vi "Read Single.vi"(0 "RS232 Port In":refnum<visa-resource-name>="COM12", 1 "Sensor Address In":string="0", 4 "Measurement Type In (Normal)":i32(ring) items=["Normal", "Concurrent", "Continuous"], 5 "CRC (False)":bool, 6 "Parameter In (0)":i32(ring) items=["0", "1", "2", "3", "4", "5", "6", "7", "8", "9"], 7 "Error In (No Error)":errorcluster, 10 "Initialize/close":bool) -> (20 "RS232 Port Out":refnum<visa-resource-name>="COM1", 21 "Sensor Address Out":string="a" caption="sensor address out", 22 "Measurements Out":dbl[](array[numeric]), 23 "Number of Measurements Out":i32, 24 "Measurement Type Out":i32(ring) items=["Normal", "Concurrent", "Continuous"], 25 "CRC Out":bool, 26 "Parameter Out":i32(ring) items=["0", "1", "2", "3", "4", "5", "6", "7", "8", "9"], 27 "Error Out":errorcluster)   [LabVIEW 2016, in "SDI-12.lvlib"]
doc: "Creates and sends a single measurement command toa sensor, and reads the measurement response(s). \n\nThe amount of data measured depends on settings of each sensor, and these settings are not ecompassed by the SDI-12 protocol.\n\nFor Normal/Concurrent Measurement Types, Read Single calls:\n1. Initiate Measurement.\n2. Wait.\n3. Fetch.\n\nFor Continuous Measurements, Read Single calls:\n1. Fetch.\n\nVisit http://www.sdi-12.org/ for more information on the SDI-12 protocol."
uses:
  SDI-12.lvlib
panel:
  out "elapsed time":dbl
  out "Max Acquisition Time (sec)":i32
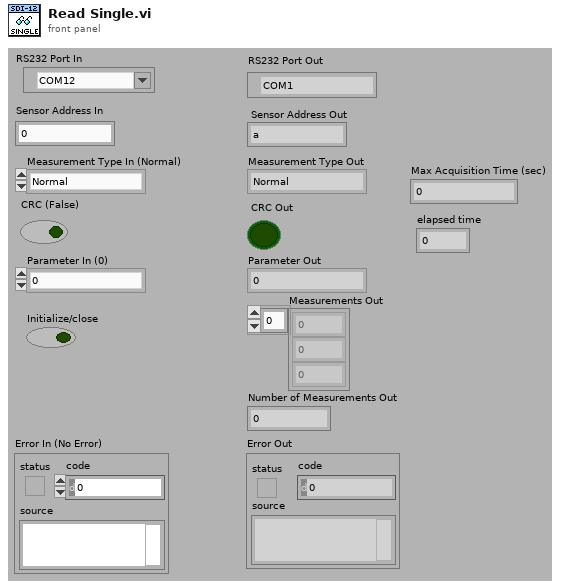
[diagram p1: front panel]
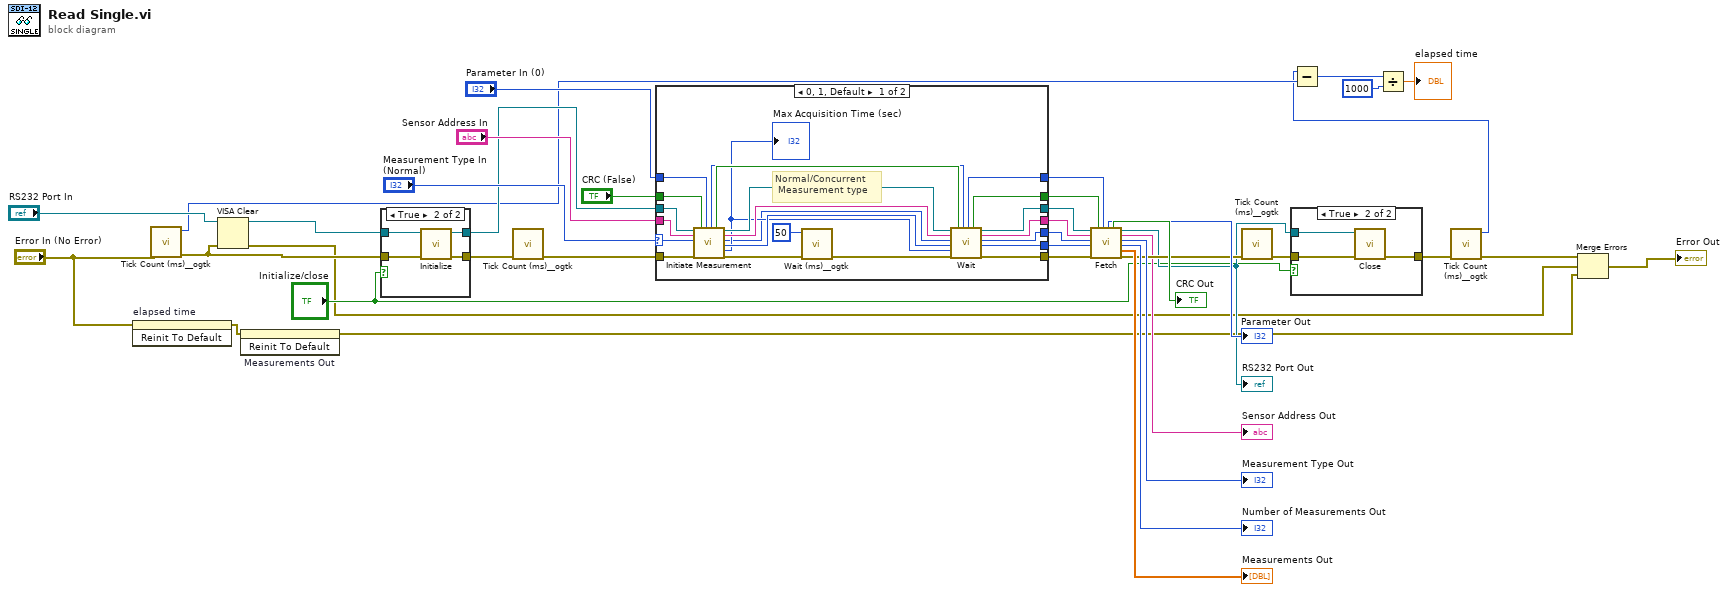
[diagram p0: block diagram]
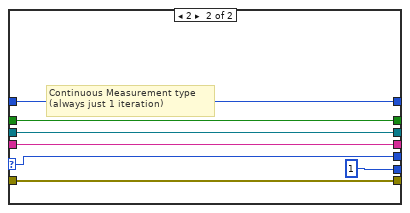
[diagram p4: hidden frame]
diagram:
  n1 = invoke on="elapsed time" class="DigNum (strict)" method="Reinit To Default"(error in="Error In (No Error)") -> (error out=w4:errorcluster)  [unwired: 2 in, 2 out]
  n2 = call <userlib>:"Tick Count (ms)__ogtk.vi"("error in (no error)"="Error In (No Error)") -> ("error out"=w6:errorcluster, "millisecond timer value"=w9:u32)  [unwired: 9 in]
  n3 = VISA Clear(VISA resource name="RS232 Port In", error in (no error)=w6) -> (VISA resource name out=w7:refnum<visa-resource-name>, error out=w1:errorcluster)
  n4 = invoke on="Measurements Out" class="Arr (strict)" method="Reinit To Default"(error in=w4) -> (error out=w2:errorcluster)  [unwired: 2 in, 2 out]
  n5 = case shown="True" "Initialize/close" {
    tunnel: w6 -> [w41 w45]
    tunnel: w7 -> [w40 w44]
    tunnel: [w41 w43] -> w17
    tunnel: [w40 w42] -> w16
    frame False {
    }
    frame True {
      n6 = call "Initialize.vi"("Error In (No Error)"=w45, "RS232 Port In"=w44) -> ("Error Out"=w43:errorcluster, "RS232 Port Out"=w42:refnum<visa-resource-name>)  [unwired: 8 in]
    }
  }
  n7 = call <userlib>:"Tick Count (ms)__ogtk.vi"("error in (no error)"=w17) -> ("error out"=w21:errorcluster)  [unwired: 9 in, 1 out]
  n8 = case shown="0, 1, Default" "Measurement Type In (Normal)" {
    selector: "Measurement Type In (Normal)" -> [w48 w70]
    tunnel: w21 -> [w68 w73]
    tunnel: "CRC (False)" -> [w67 w75]
    tunnel: "Parameter In (0)" -> [w66 w74]
    tunnel: [w61 w70] -> w22
    tunnel: [w60 1 ("Number of Measurements Out")] -> w37
    tunnel: [w59 w73] -> w36
    tunnel: [w56 w74] -> w35
    tunnel: [w55 w75] -> w34
    tunnel: w16 -> [w49 w72]
    tunnel: [w52 w72] -> w25
    tunnel: [w51 w71] -> w24
    tunnel: "Sensor Address In" -> [w50 w71]
    frame 0, 1, Default {
      # "Normal/Concurrent\n Measurement type"
      n9 = call "Initiate Measurement.vi"("RS232 Port In"=w49, "Sensor Address In"=w50, "Measurement Type In (Normal)"=w48, "Error In (No Error)"=w68, "CRC In (False)"=w67, "Parameter In (0)"=w66) -> ("Parameter Out"=w57:i32, "CRC Out"=w58:bool, "RS232 Port Out"=w64:refnum<visa-resource-name>, "Sensor Address Out"=w63:string, "Measurement Type Out"=w53:i32, "Number of Measurements"=w62:i32, "Max Acquisition Time (sec)"=w54:i32, "Error Out"=w65:errorcluster)  [unwired: 6 in]
      "Max Acquisition Time (sec)" <- w54
      n10 = call <userlib>:"Wait (ms)__ogtk.vi"("error in (no error)"=w65, "milliseconds to wait"=u32 50) -> ("error out"=w47:errorcluster)  [unwired: 8 in, 1 out]
      n11 = call "Wait.vi"("RS232 Port In"=w64, "Sensor Address In"=w63, "Measurement Type In (Normal)"=w53, "Number of Measurements In (1)"=w62, "Max Acquisition Time (0 sec)"=w54, "Error In (No Error)"=w47, "CRC (False)"=w58, "Parameter In (0)"=w57) -> ("Parameter Out"=w56:i32, "CRC Out"=w55:bool, "RS232 Port Out"=w52:refnum<visa-resource-name>, "Sensor Address Out"=w51:string, "Measurement Type Out"=w61:i32, "Number of Measurements Out"=w60:i32, "Error Out"=w59:errorcluster)  [unwired: 5 in]
    }
    frame 2 {
      # "Continuous Measurement type\n(always just 1 iteration)"
    }
  }
  n12 = call "Fetch.vi"("RS232 Port In"=w25, "Sensor Address In"=w24, "Measurement Type In (Normal)"=w22, "Number of Measurements In (1)"=w37, "Error In (No Error)"=w36, "CRC (False)"=w34, "Parameter In (0)"=w35) -> ("Parameter Out"=→"Parameter Out":i32, "CRC Out"=→"CRC Out":bool, "RS232 Port Out"=w12:refnum<visa-resource-name>, "Sensor Address Out"=→"Sensor Address Out":string, "Measurement Type Out"=→"Measurement Type Out":i32, "Number of Measurements Out"=→"Number of Measurements Out":i32, "Measurements Out"=→"Measurements Out":dbl[], "Error Out"=w27:errorcluster)  [unwired: 5 in]
  "RS232 Port Out" <- w12
  n13 = call <userlib>:"Tick Count (ms)__ogtk.vi"("error in (no error)"=w27) -> ("error out"=w14:errorcluster)  [unwired: 9 in, 1 out]
  n14 = case shown="True" "Initialize/close" {
    tunnel: [w76 w79] -> w13
    tunnel: w14 -> [w76 w78]
    tunnel: w12 -> [_ w77]
    frame False {
    }
    frame True {
      n15 = call "Close.vi"("Error In (No Error)"=w78, "RS232 Port In"=w77) -> ("Error Out"=w79:errorcluster)  [unwired: 9 in]
    }
  }
  n16 = call <userlib>:"Tick Count (ms)__ogtk.vi"("error in (no error)"=w13) -> ("error out"=w10:errorcluster, "millisecond timer value"=w8:u32)  [unwired: 9 in]
  n17 = Subtract(x=w8, y=w9) -> (x-y=w20:u32)
  n18 = Divide(x=w20, y=u32 1000) -> (x/y=→"elapsed time":dbl)
  n19 = Merge Errors(w10, w1, w2) -> (→"Error Out":errorcluster)
